vi "Set Control Limits.vi"(10 "Value Properties":T1, 11 "Control Ref":refnum<vi>) -> ()   [LabVIEW 2019, in "User Interface.lvlib"]
uses:
  User Interface.lvlib
  Packed Libraries/Audio Processing.lvlibp/Value Properties.ctl
  Packed Libraries/Audio Processing.lvlibp
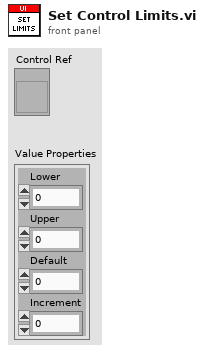
[diagram p1: front panel]
types:
  T1 = typedef "Audio Processing.lvlibp/Value Properties.ctl" = cluster{"Lower":dbl, "Upper":dbl, "Default":dbl, "Increment":dbl}
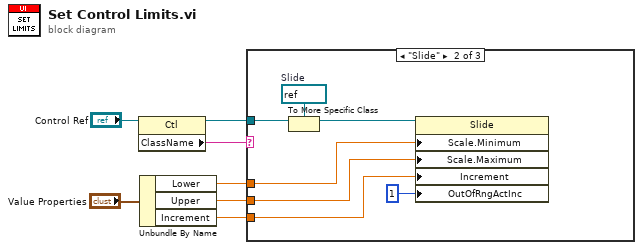
[diagram p0: block diagram]
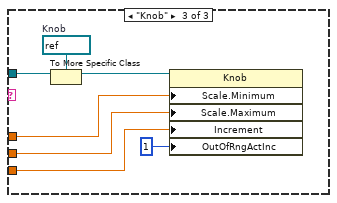
[diagram p3: hidden frame]
diagram:
  n1 = property class="Ctl"(reference="Control Ref") -> (reference out=w7:refnum<vi>, "ClassName"=w6:string)  [unwired: 1 in, 1 out]
  n2 = Unbundle By Name("Value Properties") -> ("Lower"=w3:dbl, "Upper"=w2:dbl, "Increment"=w1:dbl)
  n3 = case shown="\"Slide\"" w6 {
    tunnel: w7 -> [_ w14 w21]
    tunnel: w3 -> [_ w11 w19]
    tunnel: w2 -> [_ w10 w18]
    tunnel: w1 -> [_ w9 w16]
    frame Default {
    }
    frame "Slide" {
      w13 = refnum<vi> refnum  # Slide
      n4 = To More Specific Class(target class=w13, reference=w14) -> (specific class reference=w12:refnum<vi>)  [unwired: 1 in, 1 out]
      n5 = property class="Slide"(reference=w12, "Scale.Minimum"=w11, "Scale.Maximum"=w10, "Increment"=w9, "OutOfRngActInc"=u8 1 ("Response to Value Outside Limits:Increment")) -> ()  [unwired: 1 in, 2 out]
    }
    frame "Knob" {
      w17 = refnum<vi> refnum  # Knob
      n6 = To More Specific Class(target class=w17, reference=w21) -> (specific class reference=w20:refnum<vi>)  [unwired: 1 in, 1 out]
      n7 = property class="Knob"(reference=w20, "Scale.Minimum"=w19, "Scale.Maximum"=w18, "Increment"=w16, "OutOfRngActInc"=u8 1 ("Response to Value Outside Limits:Increment")) -> ()  [unwired: 1 in, 2 out]
    }
  }
